vi "Builtins.vi"(6 "args":string[](array[string]), 8 "error in (no error)":errorcluster, 9 "Shift?":bool, 10 "Focus":enum8{"FP", "BD"}(ring), 11 "VI Refnum":refnum<vi>) -> (0 "error out":errorcluster)   [LabVIEW 2019, in "Script.lvlib"]
doc: "Built-in script shortcuts\n\nUsage: Ctrl-Space + \"<shortcut>\" + Ctrl-S\n\nCreated by: Ryan Pacini\n\n[SCRIPT]\n--=Rename Label\n--icon=Edit VI Icon\n0=Open in File Explore\na=Arrange Diagram\naa=Align Left Edges\nas=Align Bottom Edges\nad=Align Right Edges\naw=Align Top Edges\naq=Align Vertical Centers\nae=Align Horizontal Centers\nasg=Align Controls Left and Snap to Grid\nc=Connect Pane\ncn=Cluster Size None\ncf=Cluster Size Fit\nch=Cluster Size Horizontally\ncv=Cluster Size Vertically\ndw=Distribute Top Edges\ndq=Distribute Vertical Centers\nds=Distribute Bottom Edges\ndg=Distribute Vertical Gap\nd=Distribute Vertical Compress\nda=Distribute Left Edges\nde=Distribute Horizontal Centers\ndd=Distribute Right Edges\ndh=Distribute Horizontal Gap\ndf=Distribute Horizontal Compress \ne=Resize Diagram Window\ner=Wire Error Structure\nh=Inc/Dec Buttons Hide\nhh=Inc/Dec Buttons Show\nin=Inline SubVI\nm=Merge Icon Layers\no=Reset Panel Origins\nr=Radix Hide\nrd=Radix Decimal or Normal\nrx=Radix Hex\nrb=Radix Binary or Backslash\nsc=Select Controls\nsi=Select Indicators\nsci=Select Controls and Indicators\nsn=Select None\nsg=Snap to Panel Grid\nu8=Change to U8\nu16=Change to U16\nu32=Change to U32\nu64=Change to U64\ni8=Change to I8\ni16=Change to I16\ni32=Change to I32\ni64=Change to I64\nsgl=Change to SGL\ndbl=Change to DBL\next=Change to EXT\ncsg=Change to CSG\ncdb=Change to CDB\ncxt=Change to CXT\nv=Show Label\nvv=Hide Label"
uses:
  Script.lvlib
  _builtins_arrange.ctl
  _builtins_align.ctl
  _builtins_selection.ctl
  <vilib>/numeric/LVNumericRepresentation.ctl
  _builtins_distribute.ctl
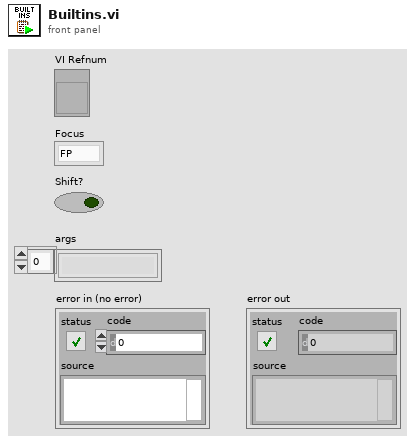
[diagram p1: front panel]
types:
  T1 = typedef "Script.lvlib/_builtins_arrange.ctl" = enum8{"left_to_right", "right_to_left"}
  T2 = typedef "Script.lvlib/_builtins_align.ctl" = enum8{"Top Edges", "Vertical Centers", "Bottom Edges", "Left Edges", "Horizontal Centers", "Right Edges"}
  T3 = typedef "Script.lvlib/_builtins_selection.ctl" = enum8{"None", "Controls", "Indicators", "Both"}
  T4 = typedef "LVNumericRepresentation.ctl" = enum32{"Extended Precision", "Double Precision", "Single Precision", "Long", "Word", "Byte", "Unsigned Long", "Unsigned Word", "Unsigned Byte", "Complex Extended", "Complex Double", "Complex Single", "Quad", "Unsigned Quad", "Fixed-Point"}
  T5 = enum8{"None", "SizeToFit", "Horizontally", "Vertically"}
  T6 = typedef "Script.lvlib/_builtins_distribute.ctl" = enum8{"Top Edges", "Vertical Centers", "Bottom Edges", "Vertical Gap", "Vertical Compress", "Left Edges", "Horizontal Centers", "Right Edges", "Horizontal Gap", "Horizontal Compress"}
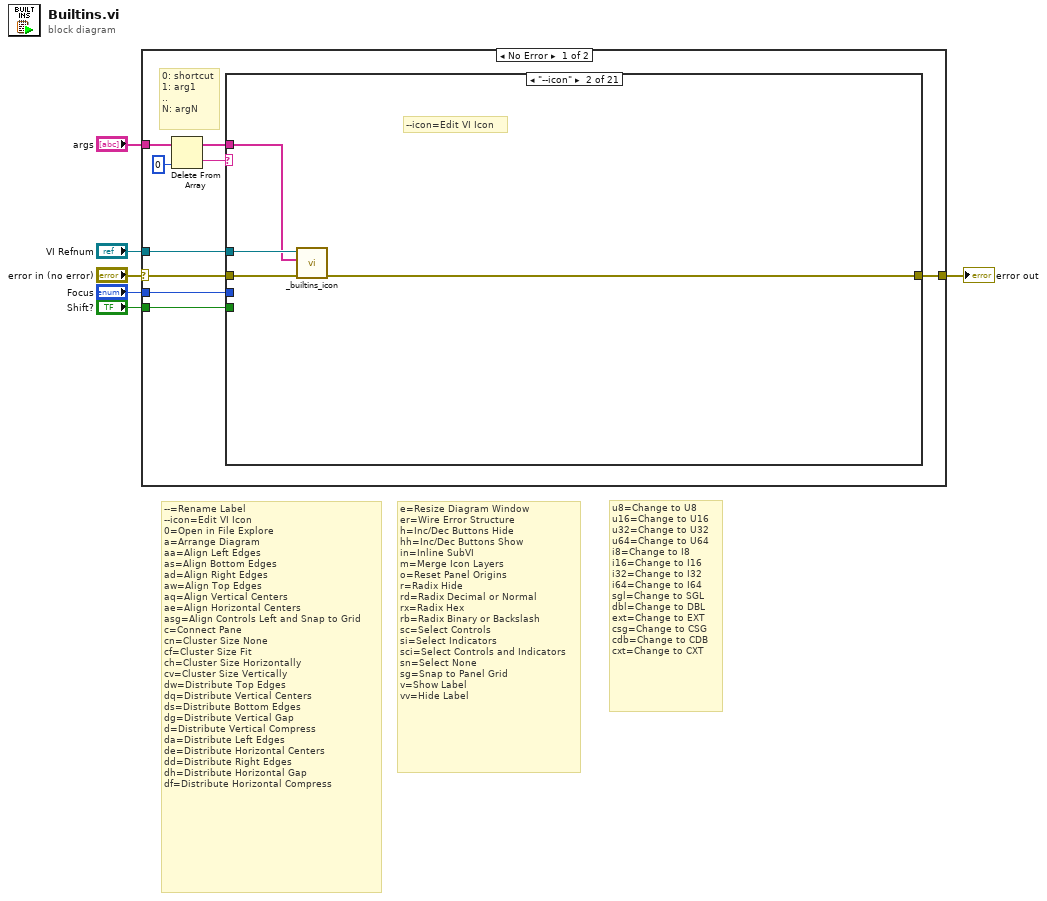
[diagram p0: block diagram]
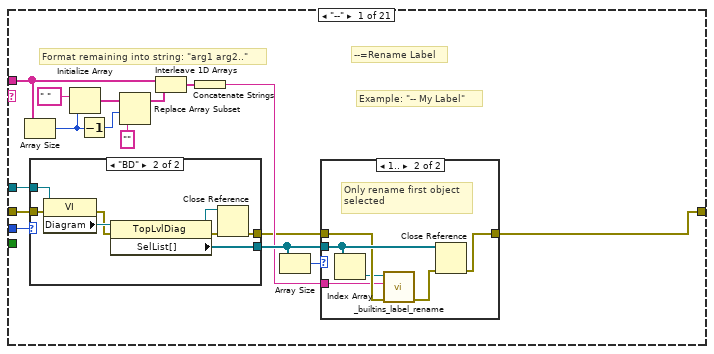
[diagram p2: hidden frame]
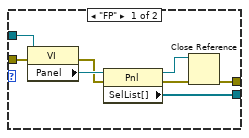
[diagram p3: hidden frame]
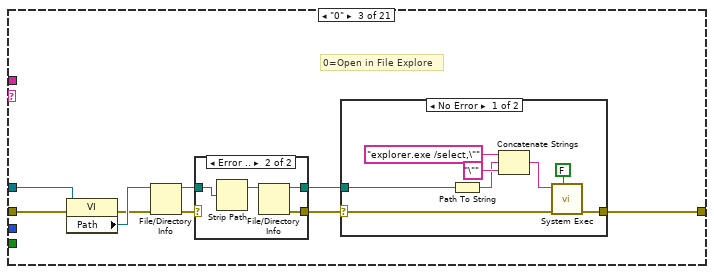
[diagram p5: hidden frame]
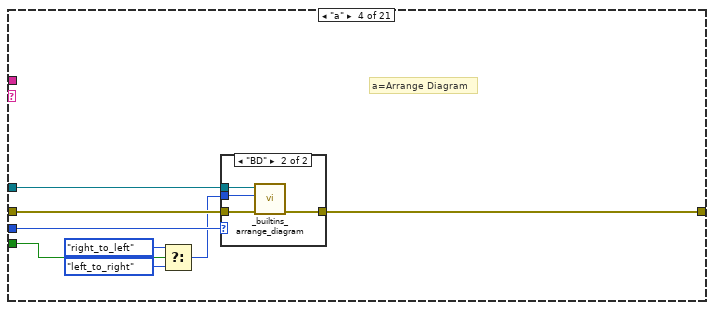
[diagram p8: hidden frame]
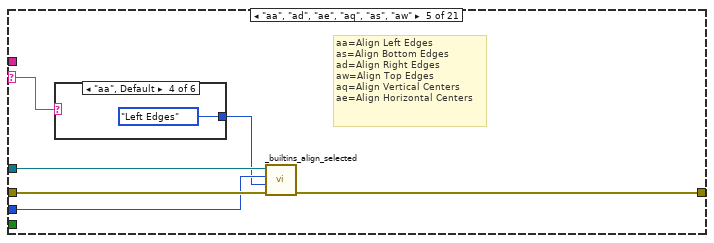
[diagram p10: hidden frame]
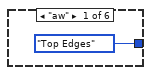
[diagram p11: hidden frame]
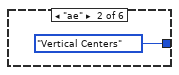
[diagram p12: hidden frame]
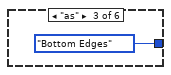
[diagram p13: hidden frame]
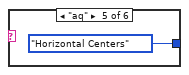
[diagram p14: hidden frame]
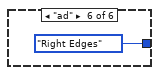
[diagram p15: hidden frame]
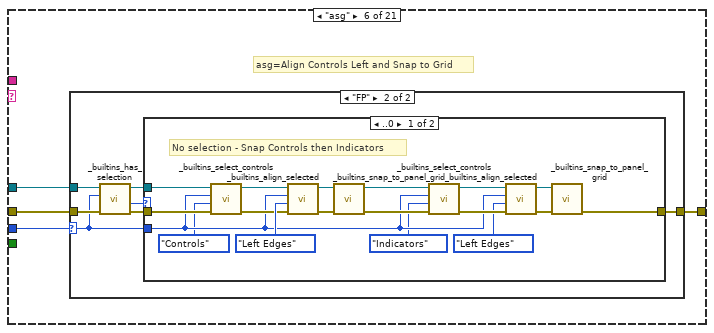
[diagram p16: hidden frame]
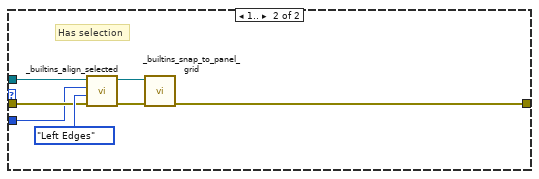
[diagram p18: hidden frame]
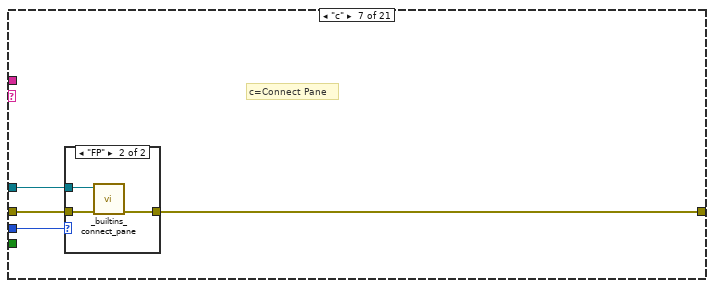
[diagram p19: hidden frame]
diagram:
  # "u8=Change to U8\nu16=Change to U16\nu32=Change to U32\nu64=Change to U64\ni8=Change to I8\ni16=Change to I16\ni32=Change to I32\ni64=Change to I64\nsgl=Change to SGL\ndbl=Change to DBL\next=Change to EXT\ncsg=Change to CSG\ncdb=Change to CDB\ncxt=Change to CXT"
  # "e=Resize Diagram Window\ner=Wire Error Structure\nh=Inc/Dec Buttons Hide\nhh=Inc/Dec Buttons Show\nin=Inline SubVI\nm=Merge Icon Layers\no=Reset Panel Origins\nr=Radix Hide\nrd=Radix Decimal or Normal\nrx=Radix Hex\nrb=Radix Binary or Backslash\nsc=Select Controls\nsi=Select Indicators\nsci=Select Controls and Indicators\nsn=Select None\nsg=Snap to Panel Grid\nv=Show Label\nvv=Hide Label"
  # "--=Rename Label\n--icon=Edit VI Icon\n0=Open in File Explore\na=Arrange Diagram\naa=Align Left Edges\nas=Align Bottom Edges\nad=Align Right Edges\naw=Align Top Edges\naq=Align Vertical Centers\nae=Align Horizontal Centers\nasg=Align Controls Left and Snap to Grid\nc=Connect Pane\ncn=Cluster Size None\ncf=Cluster Size Fit\nch=Cluster Size Horizontally\ncv=Cluster Size Vertically\ndw=Distribute Top Edges\ndq=Distribute Vertical Centers\nds=Distribute Bottom Edges\ndg=Distribute Vertical Gap\nd=Distribute Vertical Compress\nda=Distribute Left Edges\nde=Distribute Horizontal Centers\ndd=Distribute Right Edges\ndh=Distribute Horizontal Gap\ndf=Distribute Horizontal Compress"
  n1 = case shown="No Error" "error in (no error)" {
    selector: "error in (no error)" -> [w15 w453]
    tunnel: "VI Refnum" -> [w14 _]
    tunnel: "Focus" -> [w13 _]
    tunnel: "Shift?" -> [w11 _]
    tunnel: "args" -> [w10 _]
    tunnel: [w12 w453] -> w1
    frame No Error {
      # "0: shortcut\n1: arg1\n..\nN: argN"
      n2 = Delete From Array(array=w10, index=0) -> (deleted portion=w9:string, array with subset deleted=w8:string[])  [unwired: 1 in]
      n3 = case shown="\"--icon\"" w9 {
        selector: w9 -> [_ _ _ _ w96 _ _ w153 w207 w251 _ _ w279 _ _ _ w340 w385 _ w417 w451]
        tunnel: w15 -> [w23 w58 w67 w90 w101 w111 w148 w158 w212 w256 w269 w278 w284 w324 w330 w334 w345 w389 w397 w425 w452]
        tunnel: w14 -> [w22 w57 w66 w89 w100 w110 w147 w156 w210 w255 w270 w277 w282 w323 w331 w335 w343 w388 w396 w424 _]
        tunnel: w13 -> [w16 _ _ w87 w98 w109 w145 w157 w211 w254 w267 w275 w283 w321 _ w332 w344 w386 w394 w422 _]
        tunnel: [w19 w56 w65 w88 w99 w108 w146 w155 w209 w253 w268 w276 w281 w322 w329 w333 w342 w387 w395 w423 w452] -> w12
        tunnel: w11 -> [_ _ _ w86 _ _ _ _ _ _ _ _ _ _ _ _ _ _ _ _ _]
        tunnel: w8 -> [w26 w55 _ _ _ _ _ _ _ _ _ _ _ _ _ _ _ _ _ _ _]
        frame "--" {
          # "Example: \"-- My Label\""
          # "Format remaining into string: \"arg1 arg2..\""
          # "--=Rename Label"
          n4 = Array Size(array=w26) -> (size(s)=w29:i32)
          n5 = case shown="\"BD\"" w16 {
            tunnel: w23 -> [w39 w47]
            tunnel: w22 -> [w38 w46]
            tunnel: [w34 w42] -> w21
            tunnel: [w32 w40] -> w17
            frame "FP" {
              n6 = property class="VI"(reference=w38, error in=w39) -> (error out=w36:errorcluster, "Panel"=w37:refnum<vi>)  [unwired: 1 out]
              n7 = property class="Pnl"(reference=w37, error in=w36) -> (reference out=w35:refnum<vi>, error out=w33:errorcluster, "SelList[]"=w34:refnum<vi>[])
              n8 = Close Reference(reference=w35, error in (no error)=w33) -> (error out=w32:errorcluster)
            }
            frame "BD" {
              n9 = property class="VI"(reference=w46, error in=w47) -> (error out=w44:errorcluster, "Diagram"=w45:refnum<vi>)  [unwired: 1 out]
              n10 = property class="TopLvlDiag"(reference=w45, error in=w44) -> (reference out=w43:refnum<vi>, error out=w41:errorcluster, "SelList[]"=w42:refnum<vi>[])
              n11 = Close Reference(reference=w43, error in (no error)=w41) -> (error out=w40:errorcluster)
            }
          }
          n12 = Initialize Array(" ", w29) -> (w30:string[])
          n13 = Decrement(x=w29) -> (x-1=w28:i32)
          n14 = Replace Array Subset(array=w30, new element="" ("new element/subarray"), index=w28) -> (w25:string[])
          n15 = Interleave 1D Arrays(w26, w25) -> (w24:string[])
          n16 = Concatenate Strings(w24) -> (w20:string)
          n17 = Array Size(array=w21) -> (size(s)=w18:i32)
          n18 = case shown="1.." w18 {
            tunnel: w17 -> [w48 w52]
            tunnel: w21 -> [_ w54]
            tunnel: w20 -> [_ w49]
            tunnel: [w48 w53] -> w19
            frame ..0 {
              # "Nothing selected"
            }
            frame 1.. {
              # "Only rename first object\nselected"
              n19 = Index Array(array=w54) -> (element=w51:refnum<vi>)  [unwired: 1 in]
              n20 = call "_builtins_label_rename.vi"("error in (no error)"=w52, "Label"=w49, "GObject in"=w51) -> ("error out"=w50:errorcluster)  [unwired: 6 in, 2 out]
              n21 = Close Reference(reference=w54, error in (no error)=w50) -> (error out=w53:errorcluster)
            }
          }
        }
        frame "--icon" {
          # "--icon=Edit VI Icon"
          n22 = call "_builtins_icon.vi"("error in (no error)"=w58, "Args"=w55, "VI Refnum in"=w57) -> ("error out"=w56:errorcluster)  [unwired: 7 in, 1 out]
        }
        frame "0" {
          # "0=Open in File Explore"
          n23 = property class="VI"(reference=w66, error in=w67) -> (error out=w59:errorcluster, "Path"=w64:path)  [unwired: 1 out]
          n24 = File/Directory Info(path=w64, error in=w59) -> (path out=w63:path, error out=w61:errorcluster)  [unwired: 5 out]
          n25 = case shown="Error .." w61 {
            selector: w61 -> [w68 _]
            tunnel: w63 -> [w69 w73]
            tunnel: [w68 w71] -> w62
            tunnel: [w69 w70] -> w60
            frame No Error {
            }
            frame Error {
              n26 = Strip Path(path=w73) -> (stripped path=w72:path)  [unwired: 1 out]
              n27 = File/Directory Info(path=w72) -> (path out=w70:path, error out=w71:errorcluster)  [unwired: 1 in, 5 out]
            }
          }
          n28 = case shown="No Error" w62 {
            selector: w62 -> [w74 w82]
            tunnel: [w76 w82] -> w65
            tunnel: w60 -> [w75 _]
            frame No Error {
              n29 = Path To String(path=w75) -> (string=w77:string)
              n30 = Concatenate Strings("explorer.exe /select,\"" ("string"), w77, "\"" ("string")) -> (w79:string)
              n31 = call <vilib>:"System Exec.vi"("wait until completion? (T)"=FALSE, "error in (no error)"=w74, "command line"=w79) -> ("error out"=w76:errorcluster)  [unwired: 5 in, 3 out]
            }
            frame Error {
            }
          }
        }
        frame "a" {
          # "a=Arrange Diagram"
          n32 = Select(t=_builtins_arrange."right_to_left" ("Arrange"), s=w86, f=_builtins_arrange."left_to_right" ("Arrange")) -> (s? t:f=w83:T1)
          n33 = case shown="\"BD\"" w87 {
            tunnel: w90 -> [w91 w95]
            tunnel: w89 -> [_ w94]
            tunnel: w83 -> [_ w93]
            tunnel: [w91 w92] -> w88
            frame "FP" {
            }
            frame "BD" {
              n34 = call "_builtins_arrange_diagram.vi"("error in (no error)"=w95, "Arrange"=w93, "VI Refnum in"=w94) -> ("error out"=w92:errorcluster)  [unwired: 7 in, 1 out]
            }
          }
        }
        frame "aa", "ad", "ae", "aq", "as", "aw" {
          # "aa=Align Left Edges\nas=Align Bottom Edges\nad=Align Right Edges\naw=Align Top Edges\naq=Align Vertical Centers\nae=Align Horizontal Centers"
          n35 = case shown="\"aa\", Default" w96 {
            tunnel: [_builtins_align."Top Edges" ("Align Type") _builtins_align."Vertical Centers" ("Align Type") _builtins_align."Bottom Edges" ("Align Type") _builtins_align."Left Edges" ("Align Type") _builtins_align."Horizontal Centers" ("Align Type") _builtins_align."Right Edges" ("Align Type")] -> w97
            frame "aw" {
            }
            frame "ae" {
            }
            frame "as" {
            }
            frame "aa", Default {
            }
            frame "aq" {
            }
            frame "ad" {
            }
          }
          n36 = call "_builtins_align_selected.vi"("error in (no error)"=w101, "Align Type"=w97, "Panel"=w98, "VI Refnum in"=w100) -> ("error out"=w99:errorcluster)  [unwired: 6 in, 1 out]
        }
        frame "asg" {
          # "asg=Align Controls Left and Snap to Grid"
          n37 = case shown="\"FP\"" w109 {
            selector: w109 -> [_ w114]
            tunnel: w111 -> [w112 w115]
            tunnel: w110 -> [_ w116]
            tunnel: [w112 w113] -> w108
            frame "BD" {
            }
            frame "FP" {
              n38 = call "_builtins_has_selection.vi"("error in (no error)"=w115, "Focus"=w114, "VI Refnum in"=w116) -> ("error out"=w119:errorcluster, "size"=w117:i32, "VI Refnum out"=w118:refnum<vi>)  [unwired: 5 in, 1 out]
              n39 = case shown="..0" w117 {
                tunnel: [w122 w138] -> w113
                tunnel: w119 -> [w136 w140]
                tunnel: w118 -> [w137 w141]
                tunnel: w114 -> [w123 w139]
                frame ..0 {
                  # "No selection - Snap Controls then Indicators"
                  n40 = call "_builtins_select_controls.vi"("error in (no error)"=w136, "Selection"=_builtins_selection."Controls", "Focus"=w123, "VI Refnum in"=w137) -> ("error out"=w132:errorcluster, "VI Refnum out"=w131:refnum<vi>)  [unwired: 6 in]
                  n41 = call "_builtins_align_selected.vi"("error in (no error)"=w132, "Align Type"=_builtins_align."Left Edges", "Panel"=w123, "VI Refnum in"=w131) -> ("error out"=w134:errorcluster, "VI Refnum out"=w133:refnum<vi>)  [unwired: 6 in]
                  n42 = call "_builtins_snap_to_panel_grid.vi"("error in (no error)"=w134, "VI Refnum in"=w133) -> ("error out"=w124:errorcluster, "VI Refnum out"=w125:refnum<vi>)  [unwired: 8 in]
                  n43 = call "_builtins_select_controls.vi"("error in (no error)"=w124, "Selection"=_builtins_selection."Indicators", "Focus"=w123, "VI Refnum in"=w125) -> ("error out"=w129:errorcluster, "VI Refnum out"=w130:refnum<vi>)  [unwired: 6 in]
                  n44 = call "_builtins_align_selected.vi"("error in (no error)"=w129, "Align Type"=_builtins_align."Left Edges", "Panel"=w123, "VI Refnum in"=w130) -> ("error out"=w127:errorcluster, "VI Refnum out"=w128:refnum<vi>)  [unwired: 6 in]
                  n45 = call "_builtins_snap_to_panel_grid.vi"("error in (no error)"=w127, "VI Refnum in"=w128) -> ("error out"=w122:errorcluster)  [unwired: 8 in, 1 out]
                }
                frame 1.. {
                  # "Has selection"
                  n46 = call "_builtins_align_selected.vi"("error in (no error)"=w140, "Align Type"=_builtins_align."Left Edges", "Panel"=w139, "VI Refnum in"=w141) -> ("error out"=w143:errorcluster, "VI Refnum out"=w142:refnum<vi>)  [unwired: 6 in]
                  n47 = call "_builtins_snap_to_panel_grid.vi"("error in (no error)"=w143, "VI Refnum in"=w142) -> ("error out"=w138:errorcluster)  [unwired: 8 in, 1 out]
                }
              }
            }
          }
        }
        frame "c" {
          # "c=Connect Pane"
          n48 = case shown="\"FP\"" w145 {
            tunnel: w148 -> [w149 w152]
            tunnel: w147 -> [_ w151]
            tunnel: [w149 w150] -> w146
            frame "BD" {
            }
            frame "FP" {
              n49 = call "_builtins_connect_pane.vi"("error in (no error)"=w152, "VI Refnum in"=w151) -> ("error out"=w150:errorcluster)  [unwired: 8 in, 1 out]
            }
          }
        }
        frame "cdb", "csg", "cxt", "dbl", "ext", "i16", "i32", "i64", "i8", "sgl", "u16", "u32", "u64", "u8" {
          # "sgl=Change to SGL\ndbl=Change to DBL\next=Change to EXT\ncsg=Change to CSG\ncdb=Change to CDB\ncxt=Change to CXT"
          # "u8=Change to U8\nu16=Change to U16\nu32=Change to U32\nu64=Change to U64\ni8=Change to I8\ni16=Change to I16\ni32=Change to I32\ni64=Change to I64"
          n50 = case shown="\"u8\", Default" w153 {
            tunnel: [LVNumericRepresentation."Unsigned Byte" ("Representation") LVNumericRepresentation."Unsigned Word" ("Representation") LVNumericRepresentation."Unsigned Long" ("Representation") LVNumericRepresentation."Unsigned Quad" ("Representation") LVNumericRepresentation."Byte" ("Representation") LVNumericRepresentation."Word" ("Representation") LVNumericRepresentation."Long" ("Representation") LVNumericRepresentation."Quad" ("Representation") LVNumericRepresentation."Single Precision" ("Representation") LVNumericRepresentation."Double Precision" ("Representation") LVNumericRepresentation."Extended Precision" ("Representation") LVNumericRepresentation."Complex Single" ("Representation") LVNumericRepresentation."Complex Double" ("Representation") LVNumericRepresentation."Complex Extended" ("Representation")] -> w154
            frame "u8", Default {
            }
            frame "u16" {
            }
            frame "u32" {
            }
            frame "u64" {
            }
            frame "i8" {
            }
            frame "i16" {
            }
            frame "i32" {
            }
            frame "i64" {
            }
            frame "sgl" {
            }
            frame "dbl" {
            }
            frame "ext" {
            }
            frame "csg" {
            }
            frame "cdb" {
            }
            frame "cxt" {
            }
          }
          n51 = case shown="\"BD\"" w157 {
            tunnel: w158 -> [w184 w201]
            tunnel: w156 -> [w182 w199]
            tunnel: w154 -> [w180 w197]
            tunnel: [w175 w192] -> w155
            frame "BD" {
              n52 = property class="VI"(reference=w182, error in=w184) -> (error out=w183:errorcluster, "Diagram"=w181:refnum<vi>)  [unwired: 1 out]
              n53 = property class="TopLvlDiag"(reference=w181, error in=w183) -> (reference out=w177:refnum<vi>, error out=w179:errorcluster, "SelList[]"=w174:refnum<vi>[])
              n54 = for {
                tunnel: w174 -> [w189] mode=indexing
                tunnel: w180 -> [w188]
                shift-right: [w185] -> w178
                shift-left: w179 -> [w186]
                tunnel: [w187] -> w173 mode=indexing
                n55 = call "_builtins_numeric_representation.vi"("error in (no error)"=w186, "Representation"=w188, "GObject in"=w189) -> ("error out"=w185:errorcluster, "GObject out"=w187:refnum<vi>)  [unwired: 6 in, 1 out]
              }
              n56 = Close Reference(reference=w173, error in (no error)=w178) -> (error out=w176:errorcluster)
              n57 = Close Reference(reference=w177, error in (no error)=w176) -> (error out=w175:errorcluster)
            }
            frame "FP" {
              n58 = property class="VI"(reference=w199, error in=w201) -> (error out=w200:errorcluster, "Panel"=w198:refnum<vi>)  [unwired: 1 out]
              n59 = property class="Pnl"(reference=w198, error in=w200) -> (reference out=w194:refnum<vi>, error out=w196:errorcluster, "SelList[]"=w191:refnum<vi>[])
              n60 = for {
                tunnel: w191 -> [w206] mode=indexing
                tunnel: w197 -> [w205]
                shift-right: [w202] -> w195
                shift-left: w196 -> [w203]
                tunnel: [w204] -> w190 mode=indexing
                n61 = call "_builtins_numeric_representation.vi"("error in (no error)"=w203, "Representation"=w205, "GObject in"=w206) -> ("error out"=w202:errorcluster, "GObject out"=w204:refnum<vi>)  [unwired: 6 in, 1 out]
              }
              n62 = Close Reference(reference=w190, error in (no error)=w195) -> (error out=w193:errorcluster)
              n63 = Close Reference(reference=w194, error in (no error)=w193) -> (error out=w192:errorcluster)
            }
          }
        }
        frame "cf", "ch", "cn", "cv" {
          # "cn=Cluster Size None\ncf=Cluster Size Fit\nch=Cluster Size Horizontally\ncv=Cluster Size Vertically"
          n64 = case shown="\"cn\"" w207 {
            tunnel: [T5."None" ("AutoSize") T5."SizeToFit" ("AutoSize") T5."Horizontally" ("AutoSize") T5."Vertically" ("AutoSize")] -> w208
            frame "cn" {
            }
            frame "cf" {
            }
            frame "ch" {
            }
            frame "cv", Default {
            }
          }
          n65 = case shown="\"FP\"" w211 {
            tunnel: w212 -> [w228 w245]
            tunnel: w210 -> [w226 w243]
            tunnel: w208 -> [w224 w241]
            tunnel: [w219 w236] -> w209
            frame "BD" {
              n66 = property class="VI"(reference=w226, error in=w228) -> (error out=w227:errorcluster, "Diagram"=w225:refnum<vi>)  [unwired: 1 out]
              n67 = property class="TopLvlDiag"(reference=w225, error in=w227) -> (reference out=w221:refnum<vi>, error out=w223:errorcluster, "SelList[]"=w218:refnum<vi>[])
              n68 = for {
                tunnel: w218 -> [w230] mode=indexing
                tunnel: w224 -> [w229]
                shift-right: [w232] -> w222
                shift-left: w223 -> [w233]
                tunnel: [w231] -> w217 mode=indexing
                n69 = call "_builtins_cluster_autosize.vi"("error in (no error)"=w233, "AutoSize"=w229, "GObject in"=w230) -> ("error out"=w232:errorcluster, "GObject out"=w231:refnum<vi>)  [unwired: 6 in, 1 out]
              }
              n70 = Close Reference(reference=w217, error in (no error)=w222) -> (error out=w220:errorcluster)
              n71 = Close Reference(reference=w221, error in (no error)=w220) -> (error out=w219:errorcluster)
            }
            frame "FP" {
              n72 = property class="VI"(reference=w243, error in=w245) -> (error out=w244:errorcluster, "Panel"=w242:refnum<vi>)  [unwired: 1 out]
              n73 = property class="Pnl"(reference=w242, error in=w244) -> (reference out=w238:refnum<vi>, error out=w240:errorcluster, "SelList[]"=w235:refnum<vi>[])
              n74 = for {
                tunnel: w235 -> [w247] mode=indexing
                tunnel: w241 -> [w246]
                shift-right: [w249] -> w239
                shift-left: w240 -> [w250]
                tunnel: [w248] -> w234 mode=indexing
                n75 = call "_builtins_cluster_autosize.vi"("error in (no error)"=w250, "AutoSize"=w246, "GObject in"=w247) -> ("error out"=w249:errorcluster, "GObject out"=w248:refnum<vi>)  [unwired: 6 in, 1 out]
              }
              n76 = Close Reference(reference=w234, error in (no error)=w239) -> (error out=w237:errorcluster)
              n77 = Close Reference(reference=w238, error in (no error)=w237) -> (error out=w236:errorcluster)
            }
          }
        }
        frame "d", "da", "dd", "de", "df", "dg", "dh", "dq", "ds", "dw" {
          # "dw=Distribute Top Edges\ndq=Distribute Vertical Centers\nds=Distribute Bottom Edges\ndg=Distribute Vertical Gap\nd=Distribute Vertical Compress\nda=Distribute Left Edges\nde=Distribute Horizontal Centers\ndd=Distribute Right Edges\ndh=Distribute Horizontal Gap\ndf=Distribute Horizontal Compress"
          n78 = case shown="\"dw\"" w251 {
            tunnel: [_builtins_distribute."Top Edges" ("Distribute Type") _builtins_distribute."Vertical Centers" ("Distribute Type") _builtins_distribute."Bottom Edges" ("Distribute Type") _builtins_distribute."Vertical Gap" ("Distribute Type") _builtins_distribute."Vertical Compress" ("Distribute Type") _builtins_distribute."Left Edges" ("Distribute Type") _builtins_distribute."Horizontal Centers" ("Distribute Type") _builtins_distribute."Right Edges" ("Distribute Type") _builtins_distribute."Horizontal Gap" ("Distribute Type") _builtins_distribute."Horizontal Compress" ("Distribute Type")] -> w252
            frame "dw" {
            }
            frame "dq" {
            }
            frame "ds" {
            }
            frame "dg" {
            }
            frame "d", Default {
            }
            frame "da" {
            }
            frame "de" {
            }
            frame "dd" {
            }
            frame "dh" {
            }
            frame "df" {
            }
          }
          n79 = call "_builtins_distribute_selected.vi"("error in (no error)"=w256, "Distribute Type"=w252, "Panel"=w254, "VI Refnum in"=w255) -> ("error out"=w253:errorcluster)  [unwired: 6 in, 1 out]
        }
        frame "e" {
          # "e=Resize Diagram Window"
          n80 = case shown="\"BD\"" w267 {
            tunnel: w270 -> [w272 _]
            tunnel: w269 -> [w273 w274]
            tunnel: [w271 w274] -> w268
            frame "BD" {
              n81 = call "_builtins_resize_diagram_window.vi"("error in (no error)"=w273, "VI Refnum in"=w272) -> ("error out"=w271:errorcluster)  [unwired: 8 in, 1 out]
            }
            frame "FP" {
            }
          }
        }
        frame "er" {
          # "er=Wire Error Structure"
          n82 = call "_builtins_error_structure.vi"("error in (no error)"=w278, "Focus"=w275, "VI Refnum in"=w277) -> ("error out"=w276:errorcluster)  [unwired: 7 in, 1 out]
        }
        frame "h", "hh" {
          # "h=Inc/Dec Buttons Hide\nhh=Inc/Dec Buttons Show"
          n83 = case shown="\"h\", Default" w279 {
            tunnel: [enum8{"hide", "show"}."hide" ("inc/dec") enum8{"hide", "show"}."show" ("inc/dec")] -> w280
            frame "h", Default {
            }
            frame "hh" {
            }
          }
          n84 = case shown="\"BD\"" w283 {
            tunnel: w284 -> [w298 w315]
            tunnel: w282 -> [w296 w313]
            tunnel: w280 -> [w294 w311]
            tunnel: [w289 w306] -> w281
            frame "BD" {
              n85 = property class="VI"(reference=w296, error in=w298) -> (error out=w297:errorcluster, "Diagram"=w295:refnum<vi>)  [unwired: 1 out]
              n86 = property class="TopLvlDiag"(reference=w295, error in=w297) -> (reference out=w291:refnum<vi>, error out=w293:errorcluster, "SelList[]"=w288:refnum<vi>[])
              n87 = for {
                tunnel: w288 -> [w303] mode=indexing
                tunnel: w294 -> [w299]
                shift-right: [w301] -> w292
                shift-left: w293 -> [w302]
                tunnel: [w300] -> w287 mode=indexing
                n88 = call "_builtins_visible_inc_dec.vi"("error in (no error)"=w302, "inc/dec"=w299, "GObject in"=w303) -> ("error out"=w301:errorcluster, "GObject out"=w300:refnum<vi>)  [unwired: 5 in, 2 out]
              }
              n89 = Close Reference(reference=w287, error in (no error)=w292) -> (error out=w290:errorcluster)
              n90 = Close Reference(reference=w291, error in (no error)=w290) -> (error out=w289:errorcluster)
            }
            frame "FP" {
              n91 = property class="VI"(reference=w313, error in=w315) -> (error out=w314:errorcluster, "Panel"=w312:refnum<vi>)  [unwired: 1 out]
              n92 = property class="Pnl"(reference=w312, error in=w314) -> (reference out=w308:refnum<vi>, error out=w310:errorcluster, "SelList[]"=w305:refnum<vi>[])
              n93 = for {
                tunnel: w305 -> [w320] mode=indexing
                tunnel: w311 -> [w319]
                shift-right: [w317] -> w309
                shift-left: w310 -> [w318]
                tunnel: [w316] -> w304 mode=indexing
                n94 = call "_builtins_visible_inc_dec.vi"("error in (no error)"=w318, "inc/dec"=w319, "GObject in"=w320) -> ("error out"=w317:errorcluster, "GObject out"=w316:refnum<vi>)  [unwired: 5 in, 2 out]
              }
              n95 = Close Reference(reference=w304, error in (no error)=w309) -> (error out=w307:errorcluster)
              n96 = Close Reference(reference=w308, error in (no error)=w307) -> (error out=w306:errorcluster)
            }
          }
        }
        frame "in" {
          # "in=Inline SubVI"
          n97 = case shown="\"BD\"" w321 {
            tunnel: w324 -> [w325 w328]
            tunnel: w323 -> [_ w327]
            tunnel: [w325 w326] -> w322
            frame "FP" {
            }
            frame "BD" {
              n98 = call "_builtins_inline_sub_vi.vi"("error in (no error)"=w328, "VI Refnum in"=w327) -> ("error out"=w326:errorcluster)  [unwired: 8 in, 1 out]
            }
          }
        }
        frame "m" {
          # "m=Merge Icon Layers"
          n99 = call "_builtins_merge_icon_layers.vi"("error in (no error)"=w330, "VI Refnum in"=w331) -> ("error out"=w329:errorcluster)  [unwired: 8 in, 1 out]
        }
        frame "o" {
          # "o=Reset Panel Origins"
          n100 = case shown="\"FP\"" w332 {
            tunnel: w335 -> [_ w339]
            tunnel: w334 -> [w336 w338]
            tunnel: [w336 w337] -> w333
            frame "BD" {
            }
            frame "FP" {
              n101 = call "_builtins_reset_to_origin.vi"("error in (no error)"=w338, "VI Refnum in"=w339) -> ("error out"=w337:errorcluster)  [unwired: 8 in, 1 out]
            }
          }
        }
        frame "r", "rb", "rd", "rx" {
          # "r=Radix Hide\nrd=Radix Decimal or Normal\nrx=Radix Hex\nrb=Radix Binary or Backslash"
          n102 = case shown="\"rb\"" w340 {
            tunnel: [enum8{"hide", "dec", "hex", "bin"}."hide" ("radix") enum8{"hide", "dec", "hex", "bin"}."dec" ("radix") enum8{"hide", "dec", "hex", "bin"}."hex" ("radix") enum8{"hide", "dec", "hex", "bin"}."bin" ("radix")] -> w341
            frame "r" {
            }
            frame "rd", Default {
            }
            frame "rx" {
            }
            frame "rb" {
            }
          }
          n103 = case shown="\"BD\"" w344 {
            tunnel: w345 -> [w361 w378]
            tunnel: w343 -> [w359 w376]
            tunnel: w341 -> [w357 w374]
            tunnel: [w352 w369] -> w342
            frame "BD" {
              n104 = property class="VI"(reference=w359, error in=w361) -> (error out=w360:errorcluster, "Diagram"=w358:refnum<vi>)  [unwired: 1 out]
              n105 = property class="TopLvlDiag"(reference=w358, error in=w360) -> (reference out=w354:refnum<vi>, error out=w356:errorcluster, "SelList[]"=w351:refnum<vi>[])
              n106 = for {
                tunnel: w351 -> [w366] mode=indexing
                tunnel: w357 -> [w364]
                shift-right: [w363] -> w355
                shift-left: w356 -> [w365]
                tunnel: [w362] -> w350 mode=indexing
                n107 = call "_builtins_radix.vi"("error in (no error)"=w365, "radix"=w364, "GObject in"=w366) -> ("error out"=w363:errorcluster, "GObject out"=w362:refnum<vi>)  [unwired: 6 in, 1 out]
              }
              n108 = Close Reference(reference=w350, error in (no error)=w355) -> (error out=w353:errorcluster)
              n109 = Close Reference(reference=w354, error in (no error)=w353) -> (error out=w352:errorcluster)
            }
            frame "FP" {
              n110 = property class="VI"(reference=w376, error in=w378) -> (error out=w377:errorcluster, "Panel"=w375:refnum<vi>)  [unwired: 1 out]
              n111 = property class="Pnl"(reference=w375, error in=w377) -> (reference out=w371:refnum<vi>, error out=w373:errorcluster, "SelList[]"=w368:refnum<vi>[])
              n112 = for {
                tunnel: w368 -> [w383] mode=indexing
                tunnel: w374 -> [w380]
                shift-right: [w381] -> w372
                shift-left: w373 -> [w382]
                tunnel: [w379] -> w367 mode=indexing
                n113 = call "_builtins_radix.vi"("error in (no error)"=w382, "radix"=w380, "GObject in"=w383) -> ("error out"=w381:errorcluster, "GObject out"=w379:refnum<vi>)  [unwired: 6 in, 1 out]
              }
              n114 = Close Reference(reference=w367, error in (no error)=w372) -> (error out=w370:errorcluster)
              n115 = Close Reference(reference=w371, error in (no error)=w370) -> (error out=w369:errorcluster)
            }
          }
        }
        frame "sc", "sci", "si", "sn" {
          # "sc=Select Controls\nsi=Select Indicators\nsci=Select Controls and Indicators\nsn=Select None"
          n116 = case shown="\"sn\", Default" w385 {
            tunnel: [_builtins_selection."Controls" ("Selection") _builtins_selection."None" ("Selection") _builtins_selection."Indicators" ("Selection") _builtins_selection."Both" ("Selection")] -> w384
            frame "sc" {
            }
            frame "sn", Default {
            }
            frame "si" {
            }
            frame "sci" {
            }
          }
          n117 = call "_builtins_select_controls.vi"("error in (no error)"=w389, "Selection"=w384, "Focus"=w386, "VI Refnum in"=w388) -> ("error out"=w387:errorcluster)  [unwired: 6 in, 1 out]
        }
        frame "sg" {
          # "sg=Snap to Panel Grid"
          n118 = case shown="\"FP\"" w394 {
            selector: w394 -> [_ w399]
            tunnel: w397 -> [w398 w406]
            tunnel: w396 -> [_ w405]
            tunnel: [w398 w407] -> w395
            frame "BD" {
            }
            frame "FP" {
              n119 = call "_builtins_has_selection.vi"("error in (no error)"=w406, "Focus"=w399, "VI Refnum in"=w405) -> ("error out"=w403:errorcluster, "size"=w400:i32, "VI Refnum out"=w402:refnum<vi>)  [unwired: 5 in, 1 out]
              n120 = case shown="..0" w400 {
                tunnel: [w410 w415] -> w404
                tunnel: w403 -> [w411 w415]
                tunnel: w402 -> [w413 w414]
                tunnel: [w409 w414] -> w401
                tunnel: w399 -> [w412 _]
                frame ..0 {
                  # "No selection - Select All Ctrls"
                  n121 = call "_builtins_select_controls.vi"("error in (no error)"=w411, "Selection"=_builtins_selection."Both", "Focus"=w412, "VI Refnum in"=w413) -> ("error out"=w410:errorcluster, "VI Refnum out"=w409:refnum<vi>)  [unwired: 6 in]
                }
                frame 1.. {
                  # "Has selection"
                }
              }
              n122 = call "_builtins_snap_to_panel_grid.vi"("error in (no error)"=w404, "VI Refnum in"=w401) -> ("error out"=w407:errorcluster)  [unwired: 8 in, 1 out]
            }
          }
        }
        frame "v", "vv" {
          # "v=Show Label\nvv=Hide Label"
          n123 = case shown="\"BD\"" w422 {
            tunnel: w425 -> [w440 w448]
            tunnel: w424 -> [w439 w447]
            tunnel: [w435 w443] -> w421
            tunnel: [w433 w441] -> w418
            frame "FP" {
              n124 = property class="VI"(reference=w439, error in=w440) -> (error out=w437:errorcluster, "Panel"=w438:refnum<vi>)  [unwired: 1 out]
              n125 = property class="Pnl"(reference=w438, error in=w437) -> (reference out=w436:refnum<vi>, error out=w434:errorcluster, "SelList[]"=w435:refnum<vi>[])
              n126 = Close Reference(reference=w436, error in (no error)=w434) -> (error out=w433:errorcluster)
            }
            frame "BD" {
              n127 = property class="VI"(reference=w447, error in=w448) -> (error out=w445:errorcluster, "Diagram"=w446:refnum<vi>)  [unwired: 1 out]
              n128 = property class="TopLvlDiag"(reference=w446, error in=w445) -> (reference out=w444:refnum<vi>, error out=w442:errorcluster, "SelList[]"=w443:refnum<vi>[])
              n129 = Close Reference(reference=w444, error in (no error)=w442) -> (error out=w441:errorcluster)
            }
          }
          n130 = case shown="\"vv\"" w417 {
            tunnel: [enum8{"hide", "show"}."hide" ("label") enum8{"hide", "show"}."show" ("label")] -> w416
            frame "vv" {
            }
            frame "v", Default {
            }
          }
          n131 = for {
            tunnel: w421 -> [w430] mode=indexing
            tunnel: [w429] -> w420 mode=indexing
            shift-right: [w428] -> w419
            shift-left: w418 -> [w427]
            tunnel: w416 -> [w426]
            n132 = call "_builtins_visible_label.vi"("error in (no error)"=w427, "label"=w426, "GObject in"=w430) -> ("error out"=w428:errorcluster, "GObject out"=w429:refnum<vi>)  [unwired: 5 in, 2 out]
          }
          n133 = Close Reference(reference=w420, error in (no error)=w419) -> (error out=w423:errorcluster)
        }
        frame Default {
          n134 = Format Into String(format string="Script Built-Ins\n\nUnknown shortcut: %s", w451) -> (resulting string=w449:string)  [unwired: 2 in, 1 out]
          n135 = One Button Dialog(message=w449) -> ()  [unwired: 1 in, 1 out]
        }
      }
    }
    frame Error {
    }
  }
  "error out" <- w1
